vi "GetActualPosition.vi"() -> (3 "Axis_ActualPosition(°)":dbl)   [LabVIEW 2020, in "输出轴伺服.lvlib"]
uses:
  Servo_global.vi
panel:
  out "error out":errorcluster
  in  "error in (no error)":errorcluster
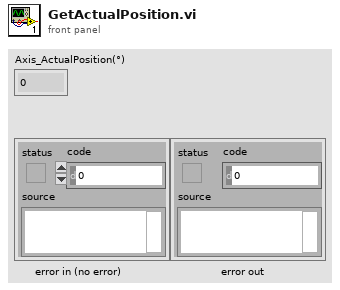
[diagram p1: front panel]
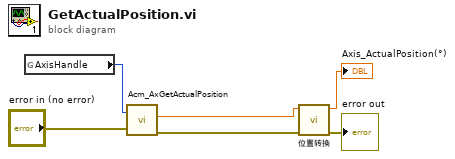
[diagram p0: block diagram]
diagram:
  n1 = global read "Servo_global.vi" "AxisHandle"() -> (w1:u32)
  n2 = call <userlib>:"Acm_AxGetActualPosition.vi"("Error Input(No Error)"="error in (no error)", "AxisHandle"=w1) -> ("Error Output"=w4:errorcluster, "Position"=w5:dbl)  [unwired: 2 out]
  n3 = call "位置转换.vi"("error in (no error)"=w4, "In"=w5) -> ("error out"=→"error out":errorcluster, "Out"=→"Axis_ActualPosition(°)":dbl)  [unwired: 8 in]
